vi "edge_scan_y.vi"(8 "error in (no error)":errorcluster, 10 "scan_y_params":T3 {"endPos" min=0 max=4000; "startPos" min=0 max=4000}, 11 "refs":T2) -> (0 "error out":errorcluster, 1 "graph":cluster{sgl[], dbl[]}, 2 "result":cluster{"maxy":sgl, "midy":sgl, "miny":sgl}, 3 "refs out":T2)   [LabVIEW 2018]
uses:
  C:/Program Files/National Instruments/LabVIEW 2018/instr.lib/IDS/ueye.NET/uEyeDotNet.dll
  <userlib>/PDamp/PDref.ctl
  <userlib>/stepper/velocity settings.ctl
  <userlib>/PDamp/channel.ctl
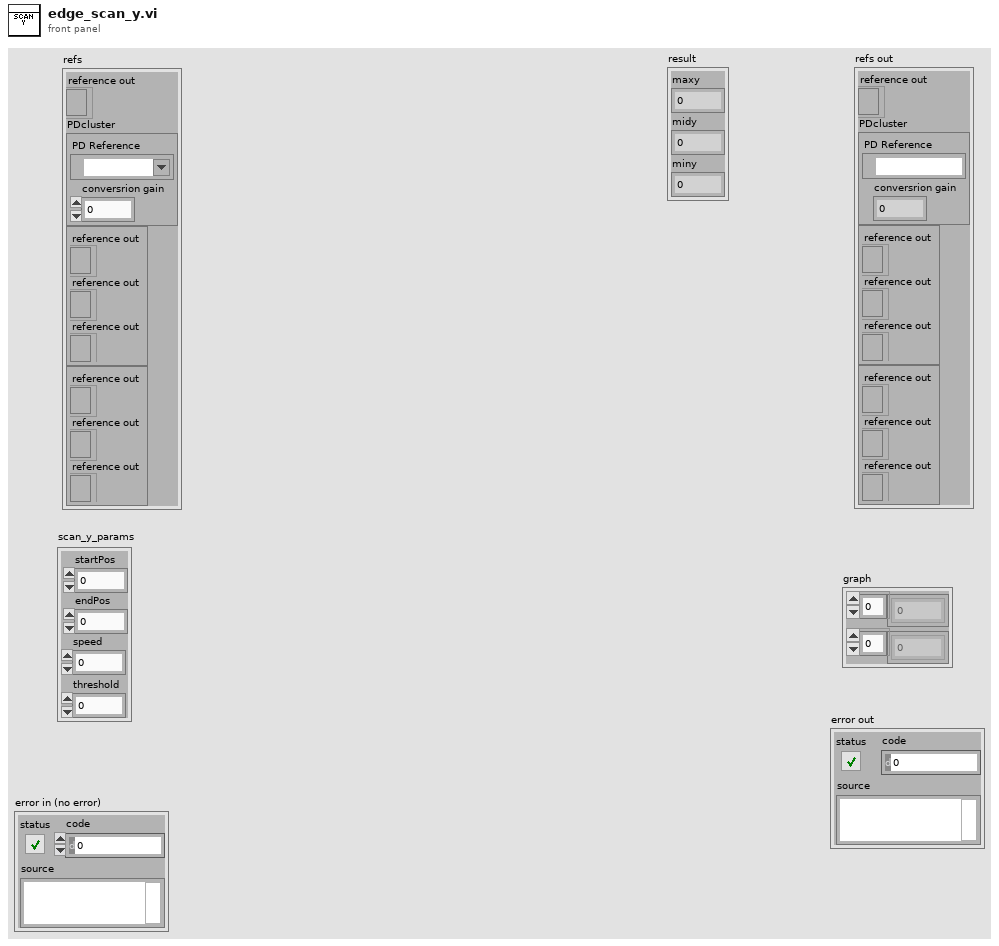
[diagram p1: front panel]
types:
  T1 = typedef "PDref.ctl" = cluster{"PD Reference":refnum<visa-resource-name>, "conversrion gain":dbl}
  T2 = cluster{"reference out":refnum<k24>, "PDcluster":T1, cluster{"reference out":refnum<k7>, "reference out":refnum<k7>, "reference out":refnum<k7>}, cluster{"reference out":refnum<k7>, "reference out":refnum<k7>, "reference out":refnum<k7>}}
  T3 = cluster{"startPos":sgl, "endPos":sgl, "speed":sgl, "threshold":sgl}
  T4 = typedef "velocity settings.ctl" = cluster{"pfMinVel":sgl, "pfAccn":sgl, "pfMaxVel":sgl}
  T5 = cluster{"reference out":refnum<k7>, "reference out":refnum<k7>, "reference out":refnum<k7>}
  T6 = typedef "channel.ctl" = enum16{"ch1", "ch2", "ch3", "ch4"}
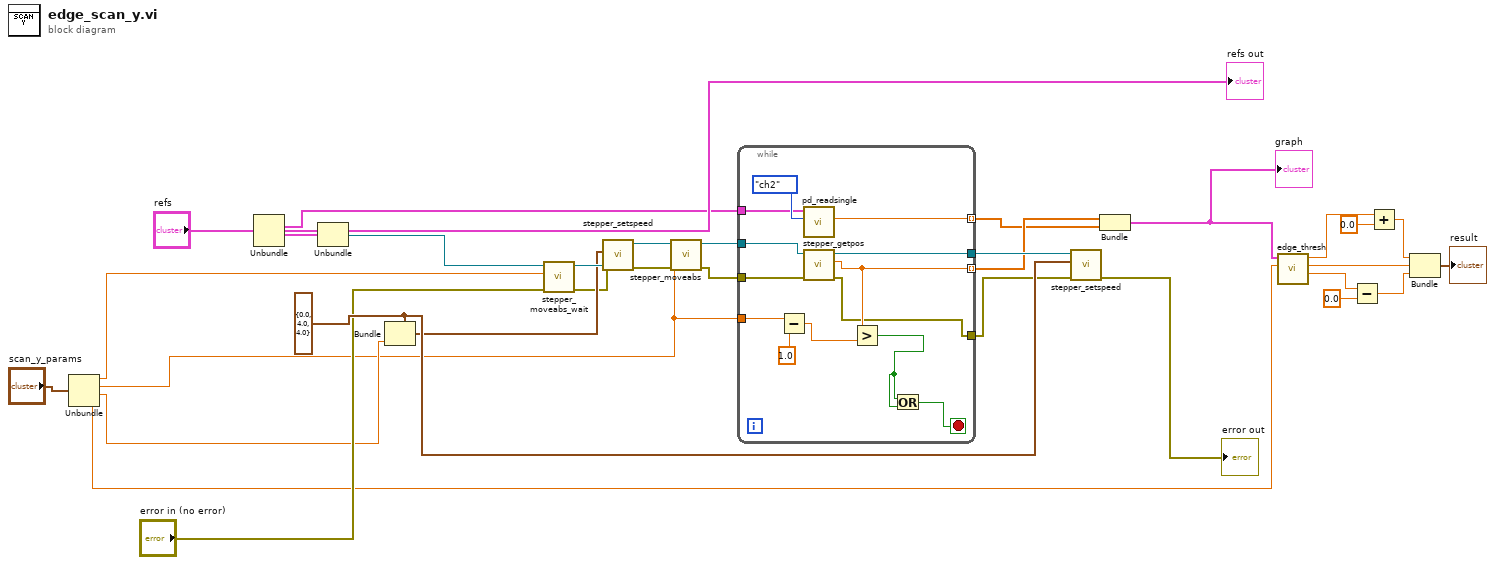
[diagram p0: block diagram]
diagram:
  w28 = T4 {"pfMinVel"=0.0, "pfAccn"=4.0, "pfMaxVel"=4.0} ("velocity parameters in")
  n1 = Unbundle("scan_y_params") -> ("startPos"=w16:sgl, "endPos"=w13:sgl, "speed"=w18:sgl, "threshold"=w9:sgl)
  n2 = Unbundle("refs") -> ("PDcluster"=w15:T1, w31:T5)  [unwired: 2 out]
  n3 = Unbundle(w31) -> ("reference out"=w30:refnum<k7>)  [unwired: 2 out]
  n4 = Bundle(cluster=w28, "pfMaxVel"=w18) -> (w25:T4)  [unwired: 2 in]
  n5 = call <userlib>:"stepper_moveabs_wait.vi"("error in (no error)"="error in (no error)", "fAbsPos[µm]"=w16, "reference"=w30) -> ("error out"=w24:errorcluster, "reference out"=w29:refnum<k7>)  [unwired: 7 in]
  n6 = call <userlib>:"stepper_setspeed.vi"("error in (no error)"=w24, "velocity parameters in"=w25, "reference"=w29) -> ("error out"=w23:errorcluster, "reference out"=w26:refnum<k7>)  [unwired: 6 in, 1 out]
  n7 = call <userlib>:"stepper_moveabs.vi"("error in (no error)"=w23, "fAbsPos[µm]"=w13, "reference"=w26) -> ("error out"=w22:errorcluster, "reference out"=w17:refnum<k7>)  [unwired: 7 in]
  n8 = while {
    tunnel: [w44] -> w11 mode=indexing
    tunnel: [w42] -> w12 mode=indexing
    tunnel: [w40] -> w27
    tunnel: [w38] -> w21
    tunnel: w22 -> [w36]
    tunnel: w17 -> [w35]
    tunnel: w15 -> [w34]
    tunnel: w13 -> [w33]
    stop <- w39 stop-if-true
    n9 = Subtract(x=w33, y=sgl 1.0) -> (x-y=w41:sgl)
    n10 = call <userlib>:"pd_readsingle.vi"("PDcluster in"=w34, "channel"=channel."ch2") -> ("photocurrent"=w44:dbl)  [unwired: 6 in, 2 out]
    n11 = call <userlib>:"stepper_getpos.vi"("error in (no error)"=w36, "reference"=w35) -> ("error out"=w38:errorcluster, "pfPosition[µm]"=w42:sgl, "reference out"=w40:refnum<k7>)  [unwired: 7 in]
    n12 = Greater?(x=w42, y=w41) -> (0:w37:bool)
    n13 = Or(x=w37, y=w37) -> (x .or. y?=w39:bool)
  }
  n14 = call <userlib>:"stepper_setspeed.vi"("error in (no error)"=w21, "velocity parameters in"=w28, "reference"=w27) -> ("error out"=→"error out":errorcluster)  [unwired: 6 in, 2 out]
  n15 = Bundle(w12, w11) -> (w10:cluster{sgl[], dbl[]})  [unwired: 1 in]
  "graph" <- w10
  n16 = call "edge_thresh.vi"("threshold"=w9, "input cluster"=w10) -> ("miny"=w2:sgl, "midy"=w8:sgl, "maxy"=w6:sgl)  [unwired: 7 in]
  n17 = Subtract(x=w2, y=sgl 0.0) -> (x-y=w1:sgl)
  n18 = Add(x=w6, y=sgl 0.0) -> (x+y=w4:sgl)
  n19 = Bundle(w4, "midy"=w8, w1) -> (→"result":cluster{sgl, "midy":sgl, sgl})  [unwired: 1 in]
  "refs out" <- "refs"
